vi "Kikusui PLZ-Clear Protection Alarm.vi"(8 "error in":errorcluster, 11 "Kikusui PLZ Setting In":T1={"VISA Resource Name"="", "Baud Rate"=19200, "Stop Bits"=20, "Wait For Read(ms)"=0} {"Stop Bits" items=["1.0"=10, "2.0"=20]; "Baud Rate" items=["2400"=2400, "4800"=4800, "9600"=9600, "19200"=19200]}) -> (0 "error out":errorcluster, 3 "Kikusui PLZ Setting Out":T1={"VISA Resource Name"="", "Baud Rate"=19200, "Stop Bits"=20, "Wait For Read(ms)"=0} {"Stop Bits" items=["1.0"=10, "2.0"=20]; "Baud Rate" items=["2400"=2400, "4800"=4800, "9600"=9600, "19200"=19200]})   [LabVIEW 2018]
uses:
  Data Def/Kikusui PLZ-Setting.ctl
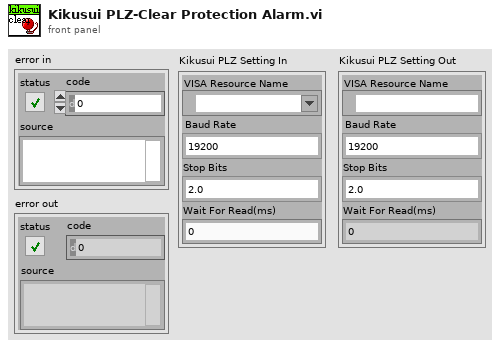
[diagram p1: front panel]
types:
  T1 = typedef "Kikusui PLZ-Setting.ctl" = cluster{"VISA Resource Name":refnum<visa-resource-name>, "Baud Rate":u32, "Stop Bits":u16, "Wait For Read(ms)":u32}
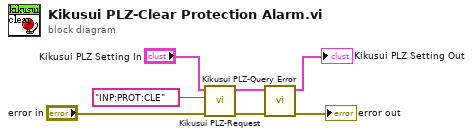
[diagram p0: block diagram]
diagram:
  n1 = call "Kikusui PLZ-Request.vi"("error in"="error in", "Command"="INP:PROT:CLE" ("write buffer"), "Kikusui PLZ Setting In"="Kikusui PLZ Setting In") -> ("error out"=w6:errorcluster, "Kikusui PLZ Setting Out"=w2:T1)  [unwired: 6 in, 1 out]
  n2 = call "Kikusui PLZ-Query Error.vi"("error in"=w6, "Kikusui PLZ Setting In"=w2) -> ("error out"=→"error out":errorcluster, "Kikusui PLZ Setting Out"=→"Kikusui PLZ Setting Out":T1)  [unwired: 8 in]
